vi "Get_TriggerOutput_Source.vi"(8 "error in (no error)":errorcluster, 11 ".NET Reference in":refnum<k24>) -> (0 "error out":errorcluster, 2 "mode":enum16{"Wavelength", "Time", ""}(ring), 3 ".NET Reference out":refnum<k24>)   [LabVIEW 2017]
uses:
  D:/test/FULLband-sts/Fullband_Sample/DLL/InstrumentDLL.dll
  DLL/InstrumentDLL.dll
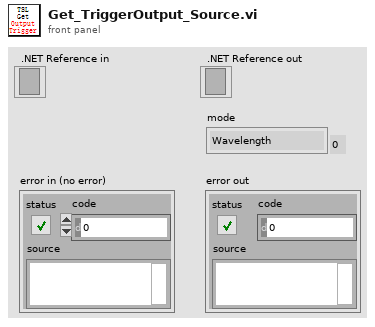
[diagram p1: front panel]
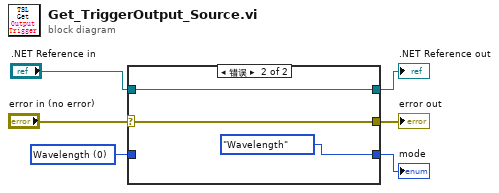
[diagram p0: block diagram]
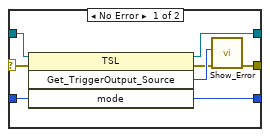
[diagram p2: hidden frame]
diagram:
  w2 = 0 items=["Wavelength", "Time"] ("mode")
  n1 = case shown="错误" "error in (no error)" {
    selector: "error in (no error)" -> [w7 w17]
    tunnel: [w8 w17] -> w6
    tunnel: [w14 w16] -> w5
    tunnel: ".NET Reference in" -> [w13 w16]
    tunnel: [w12 enum16{"Wavelength", "Time", ""}."Wavelength" ("mode")] -> w3
    tunnel: w2 -> [w11 _]
    frame No Error {
      n2 = invoke on="调用节点" class="TSL" method="Get_TriggerOutput_Source"(reference=w13, error in=w7, "mode"=w11) -> (reference out=w14:refnum<k24>, error out=w9:errorcluster, "Get_TriggerOutput_Source"=w10:i32, "mode"=w12:i32)  [unwired: 1 in]
      n3 = call "Show_Error.vi"("error in (no error)"=w9, "Error"=w10) -> ("error out"=w8:errorcluster)  [unwired: 9 in]
    }
    frame Error {
    }
  }
  "error out" <- w6
  ".NET Reference out" <- w5
  "mode" <- w3
